vi "Find Custom Device by Name.vi"(8 "error in (no error)":errorcluster, 10 "Name":string, 11 "Target in":refnum<k24>) -> (0 "error out":errorcluster, 2 "Custom Device":refnum<k24>, 3 "Target out":refnum<k24>)   [LabVIEW 2017, in "Switch Scripting.lvlib"]
uses:
  Switch Scripting.lvlib
  NationalInstruments.VeriStand.SystemDefinitionAPI
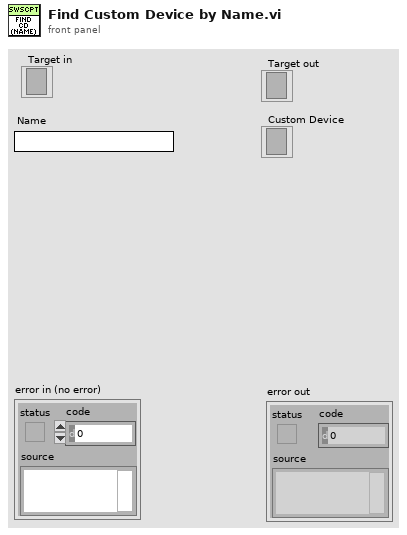
[diagram p1: front panel]
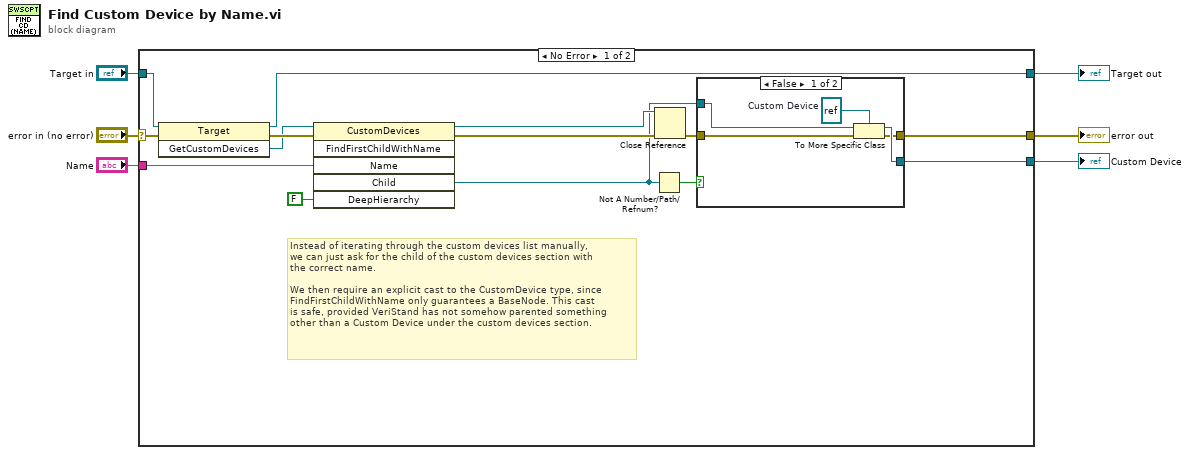
[diagram p0: block diagram]
diagram:
  n1 = case shown="No Error" "error in (no error)" {
    selector: "error in (no error)" -> [w20 w28]
    tunnel: [w12 w28] -> w6
    tunnel: "Target in" -> [w19 w27]
    tunnel: [w10 w27] -> w3
    tunnel: "Name" -> [w15 _]
    tunnel: [w7 _] -> w1
    frame No Error {
      # "Instead of iterating through the custom devices list manually,\nwe can just ask for the child of the custom devices section with\nthe correct name.\n\nWe then require an explicit cast to the CustomDevice type, since\nFindFirstChildWithName only guarantees a BaseNode. This cast\nis safe, provided VeriStand has not somehow parented something\nother than a Custom Device under the custom devices section."
      n2 = invoke class="Target" method="GetCustomDevices"(reference=w19, error in=w20) -> (reference out=w10:refnum<k24>, error out=w18:errorcluster, "GetCustomDevices"=w17:refnum<k24>)  [unwired: 1 in]
      n3 = invoke class="CustomDevices" method="FindFirstChildWithName"(reference=w17, error in=w18, "Name"=w15, "DeepHierarchy"=FALSE) -> (reference out=w14:refnum<k24>, error out=w13:errorcluster, "Child"=w9:refnum<k24>)  [unwired: 2 in, 3 out]
      n4 = Not A Number/Path/Refnum?(number/path/refnum=w9) -> (NaN/Path/Refnum?=w8:bool)
      n5 = Close Reference(reference=w14, error in (no error)=w13) -> (error out=w11:errorcluster)
      n6 = case shown="False" w8 {
        tunnel: [w24 _] -> w7
        tunnel: [w23 w26] -> w12
        tunnel: w11 -> [w22 w26]
        tunnel: w9 -> [w21 _]
        frame False {
          w25 = refnum<k24> refnum  # Custom Device
          n7 = To More Specific Class(target class=w25, reference=w21, error in=w22) -> (specific class reference=w24:refnum<k24>, error out=w23:errorcluster)
        }
        frame True {
        }
      }
    }
    frame Error {
    }
  }
  "Target out" <- w3
  "error out" <- w6
  "Custom Device" <- w1
